vi "Create report name.vi"(8 "error in (no error)":errorcluster, 11 "SAP ID":string) -> (0 "error out":errorcluster, 3 "filename":string)   [LabVIEW 2018, in "Application.lvlib"]
uses:
  Application.lvlib
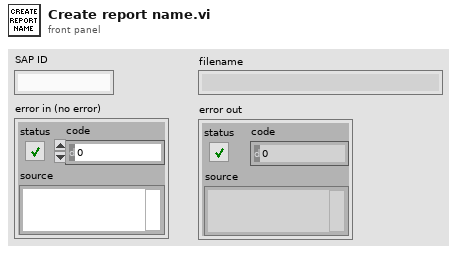
[diagram p1: front panel]
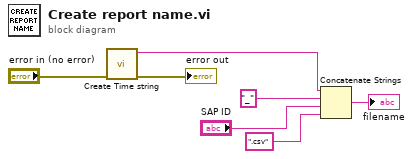
[diagram p0: block diagram]
diagram:
  n1 = call "Create Time string.vi"("error in (no error)"="error in (no error)") -> ("error out"=→"error out":errorcluster, "Timestr"=w4:string)  [unwired: 9 in]
  n2 = Concatenate Strings(w4, "_", "SAP ID", ".csv") -> (→"filename":string)
